vi "setArmMotor.vi"(9 "Boolean 2":bool, 10 "Boolean":bool, 11 "Arm Pickup":bool) -> (3 "f":dbl)   [LabVIEW 2014]
uses:
  LabVIEW Data/2015 Beta Robot Project/Robot Global Data.vi
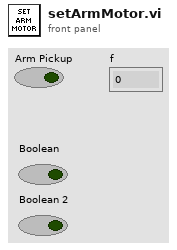
[diagram p1: front panel]
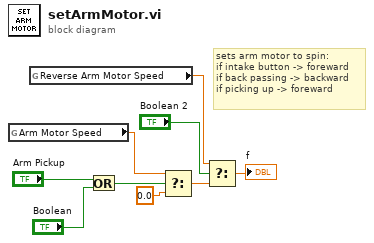
[diagram p0: block diagram]
diagram:
  # "sets arm motor to spin:\nif intake button -> foreward\nif back passing -> backward\nif picking up -> foreward"
  n1 = global read "Robot Global Data.vi" "Arm Motor Speed"() -> (w5:dbl)
  n2 = global read "Robot Global Data.vi" "Reverse Arm Motor Speed"() -> (w1:dbl)
  n3 = Or(x="Arm Pickup", y="Boolean") -> (x .or. y?=w6:bool)
  n4 = Select(t=w5, s=w6, f=0.0) -> (s? t:f=w2:dbl)
  n5 = Select(t=w1, s="Boolean 2", f=w2) -> (s? t:f=→"f":dbl)
